vi "Show Open VIs Main Dialog.vi"(8 "error in (no error)":errorcluster) -> (0 "error out":errorcluster)   [LabVIEW 2011]
doc: "This VI will show a dialog of all the VIs that are currently open. Then this VI will allow you to select one to open the front panel, block diagram, or abort.\n\nDeveloped by Brian Hoover brian@brian-hoover.com"
uses:
  VI Data Type.ctl
  <vilib>/picture/picture.llb/imagedata.ctl
  <vilib>/Utility/miscctls.llb/LVBoundsTypeDef.ctl
  <userlib>/_OpenG.lib/array/array.llb/Conditional Auto-Indexing Tunnel (Variant)__ogtk.vi
  <userlib>/_OpenG.lib/file/file.llb/Strip Path - Traditional__ogtk.vi
panel:
  in  "n":dbl
  in  "Refresh":bool
  out "2D Picture":picture
  out "VI Name":string
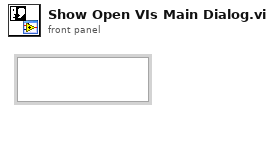
[diagram p1: front panel]
types:
  T1 = typedef "LVBoundsTypeDef.ctl" = cluster{"Width":u32, "Height":u32}
  T2 = typedef "VI Data Type.ctl" = cluster{"App Refnum":refnum<vi>, "VI Name":string, "VI Icon":T3}
  T3 = typedef "imagedata.ctl" = cluster{"image type":i32, "image depth":i32, "image":u8[], "mask":u8[], "colors":u32[], "Rectangle":cluster{"left":i16, "top":i16, "right":i16, "bottom":i16}}
  T4 = cluster{"Resize?":bool, "All VI Data":T2[], "Last Selected VI":T2, "Cell Bounds":T1, "# of Rows":i32, "# of Columns":i32, "Original Picture":picture}
  T5 = cluster{"Width":i16, "Style":enum32{"Solid", "Dash", "Dot", "DashDot", "DashDotDot"}}
  T6 = enum32{"Invalid", "Standard", "Closed", "Hidden", "Minimized", "Maximized"}
  T7 = typedef "LVPoint32TypeDef.ctl" = cluster{"Horizontal":i32, "Vertical":i32}
  T8 = cluster{"Width":u32, "Height":u32, "Width":u32, "Height":u32}
  T9 = cluster{"Shift":bool, "Ctrl":bool, "Alt":bool, "Cmd":bool, "Opt":bool}
  T10 = enum32{"Bad", "Idle", "Run top level", "Running"}
  T11 = typedef "VIMemory VI info.ctl" = cluster{"Project":string, "ComputingNode":string, "VI Name":string, "App Refnum":refnum<vi>}
  T12 = typedef "LVRectTypeDef.ctl" = cluster{"left":i16, "top":i16, "right":i16, "bottom":i16}
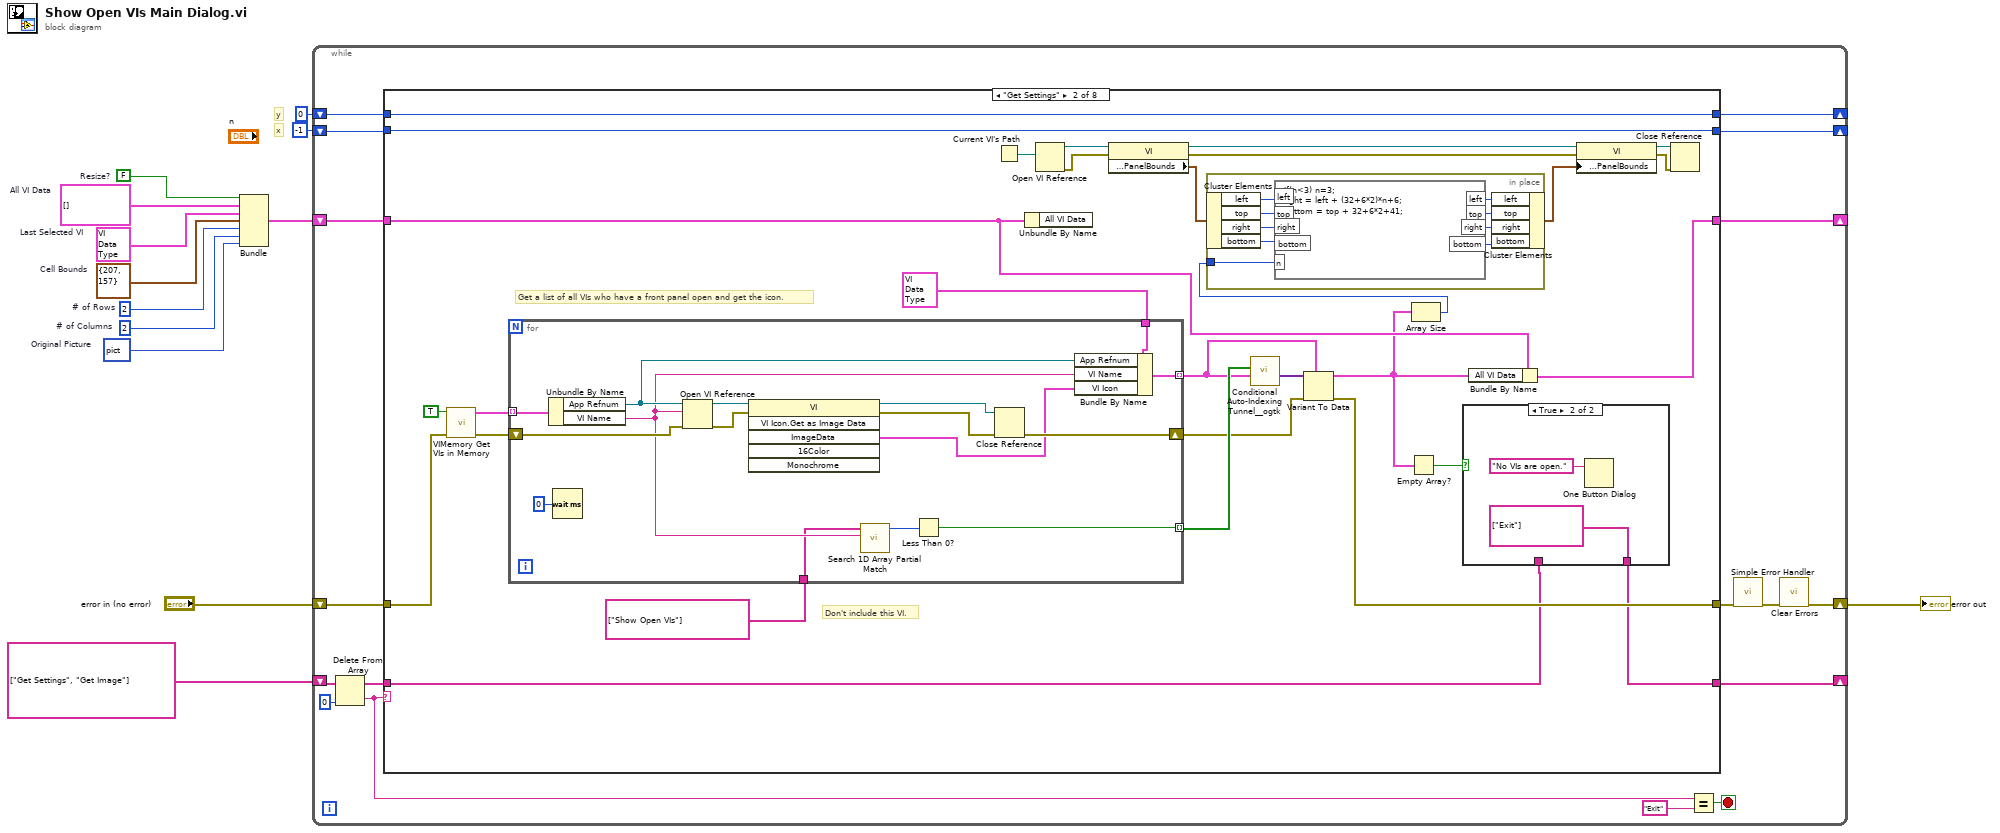
[diagram p0: block diagram]
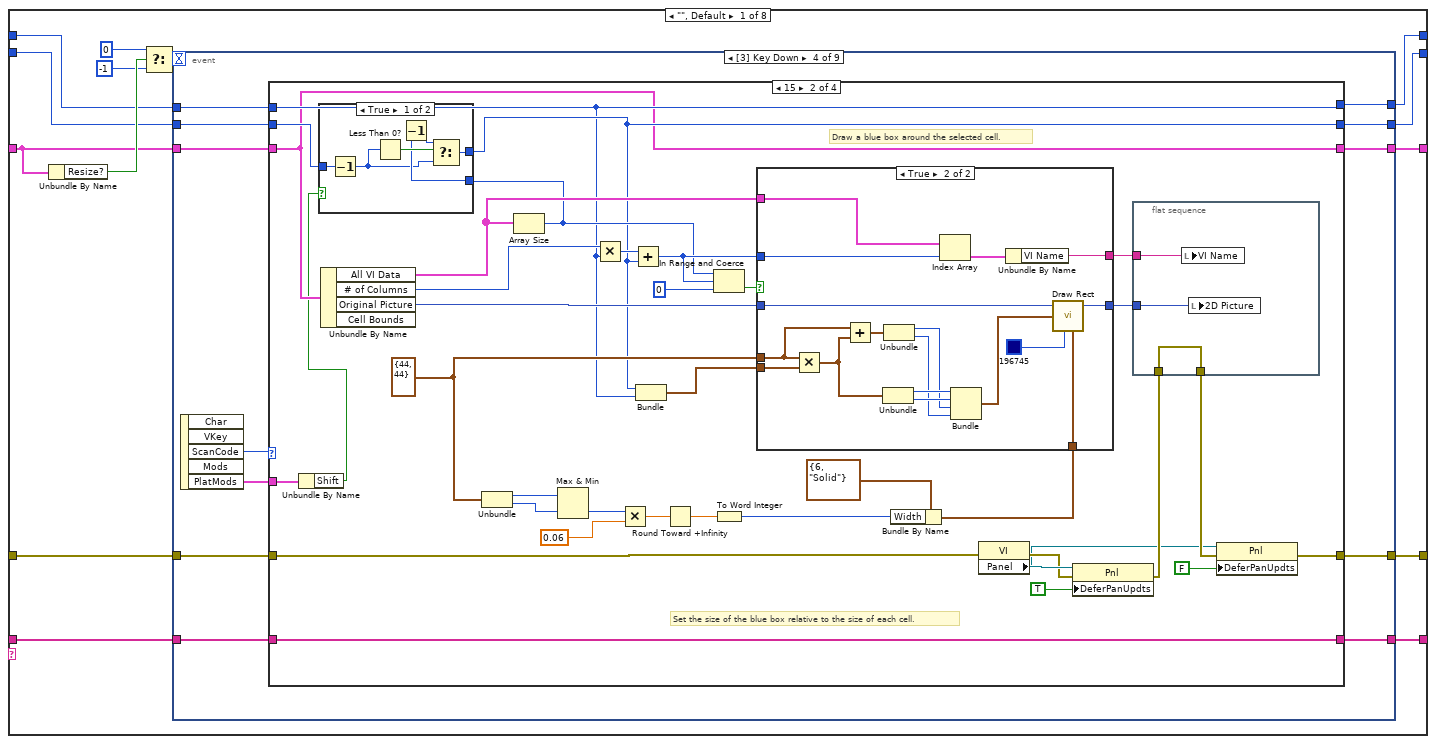
[diagram p2: hidden frame]
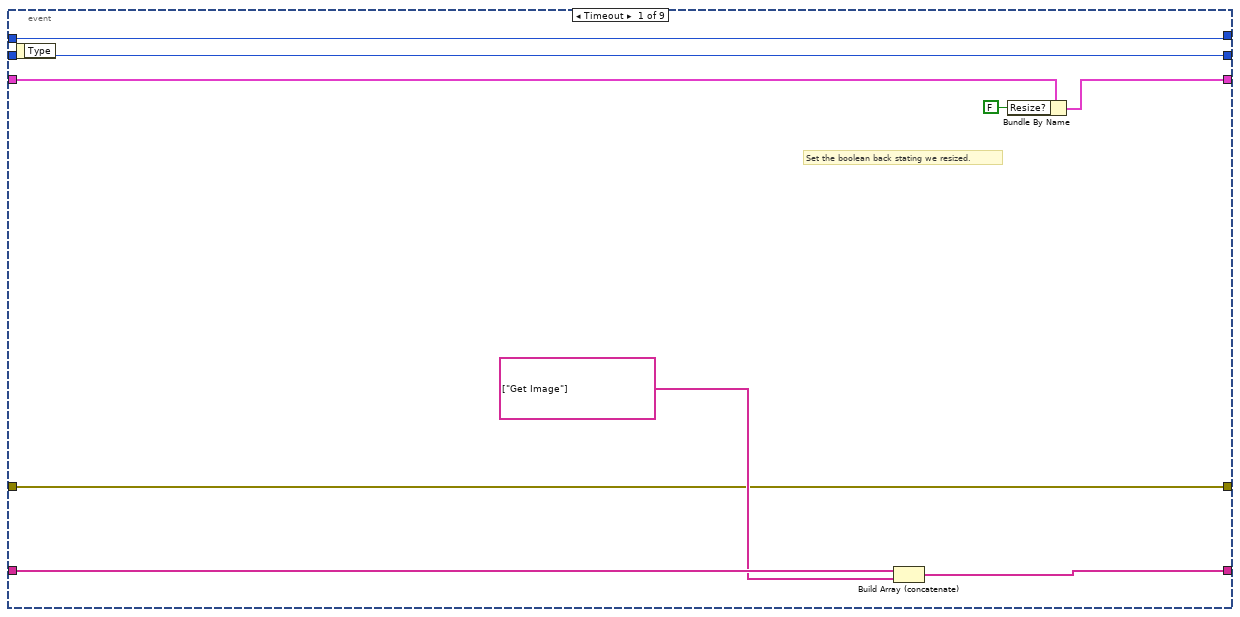
[diagram p3: hidden frame]
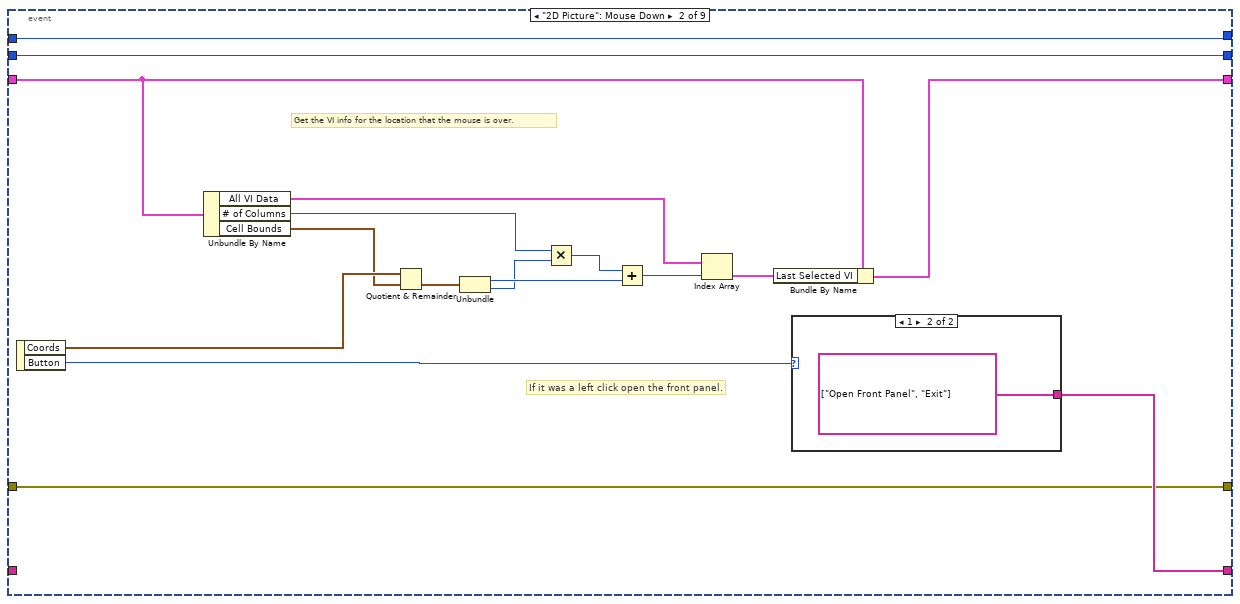
[diagram p4: hidden frame]
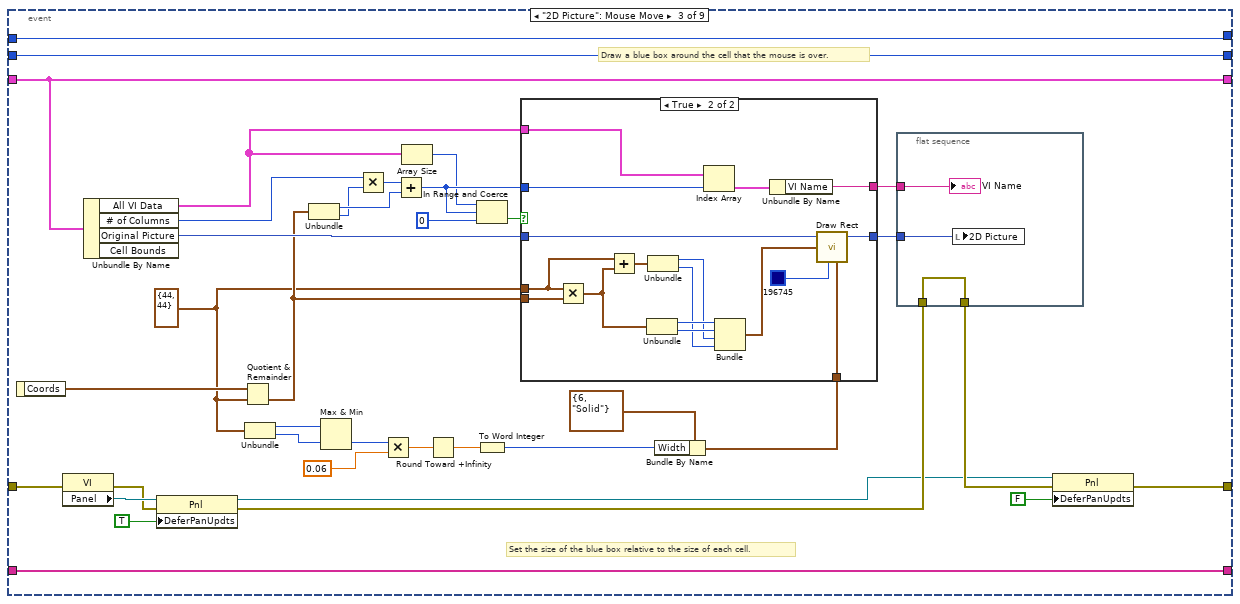
[diagram p6: hidden frame]
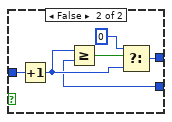
[diagram p9: hidden frame]
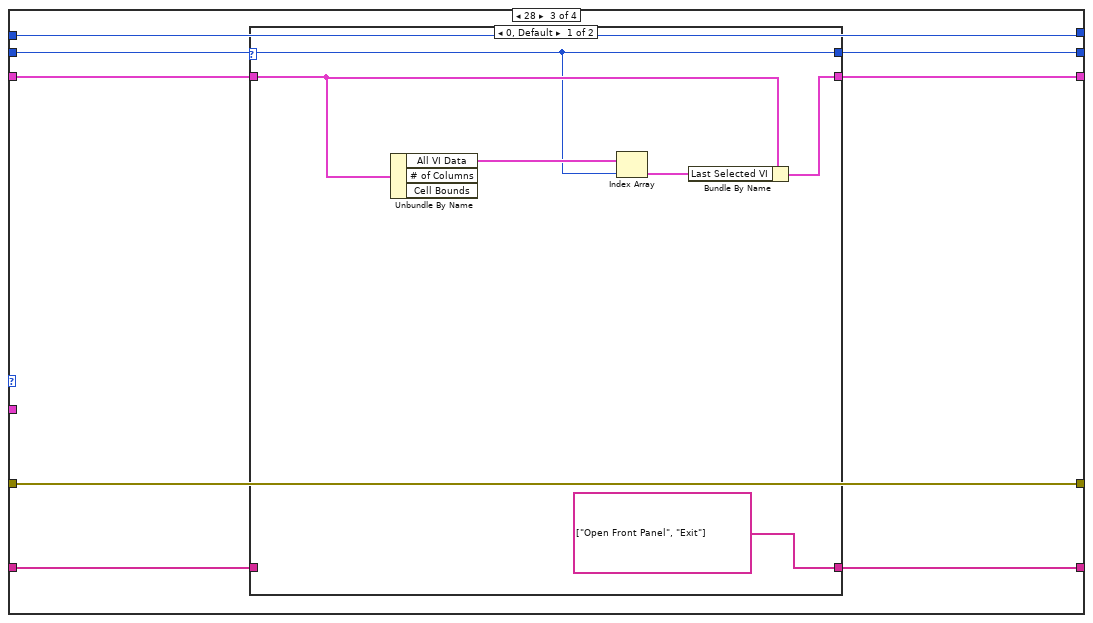
[diagram p11: hidden frame]
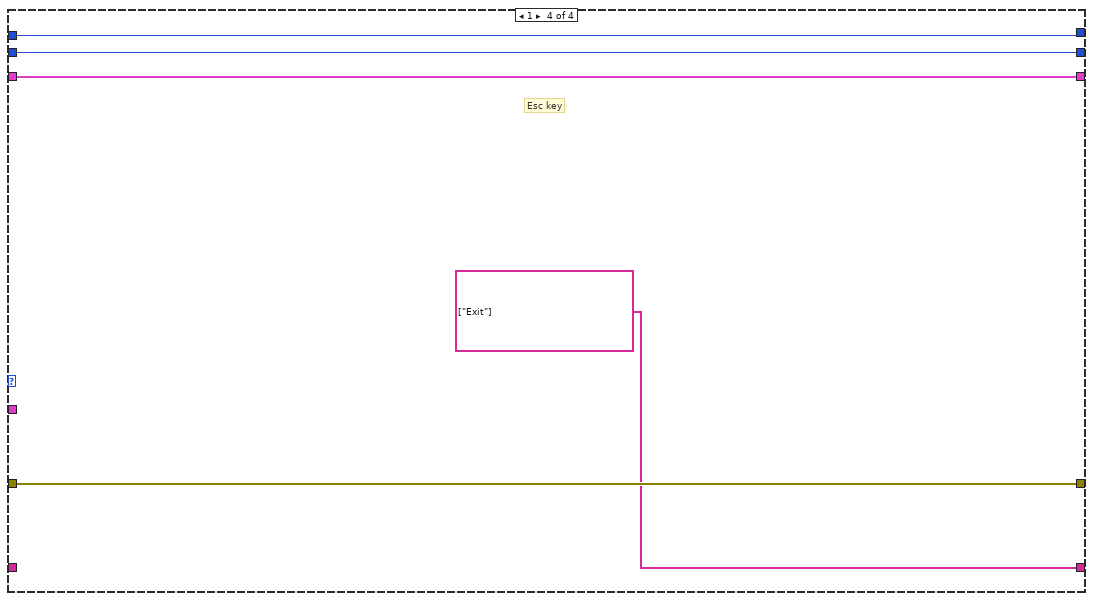
[diagram p13: hidden frame]
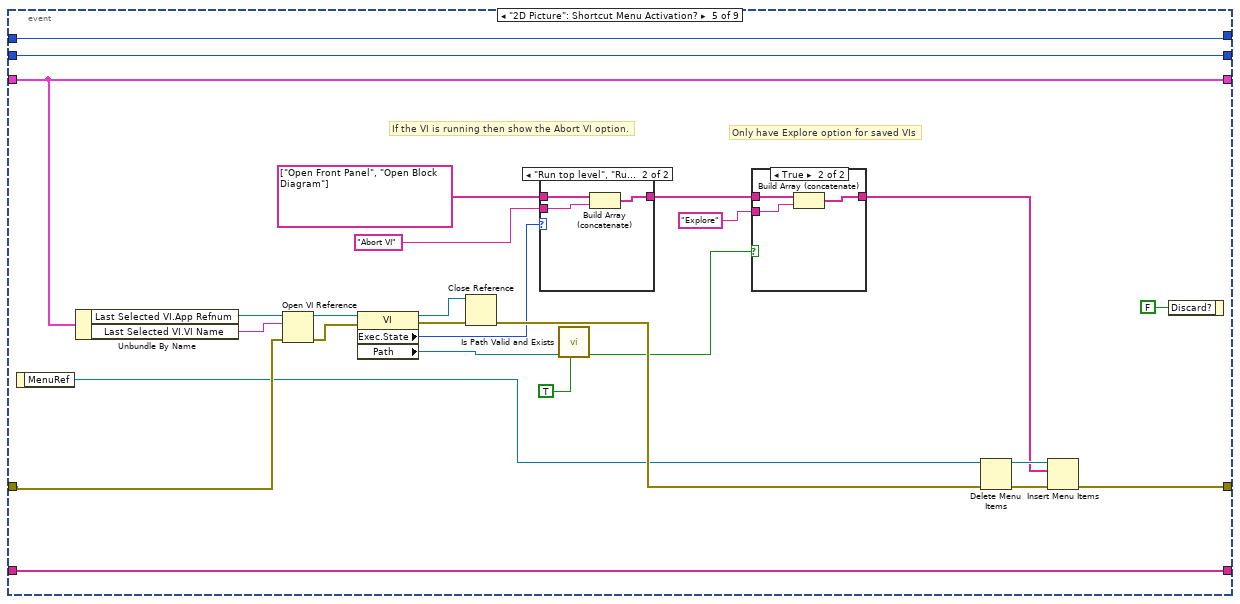
[diagram p14: hidden frame]
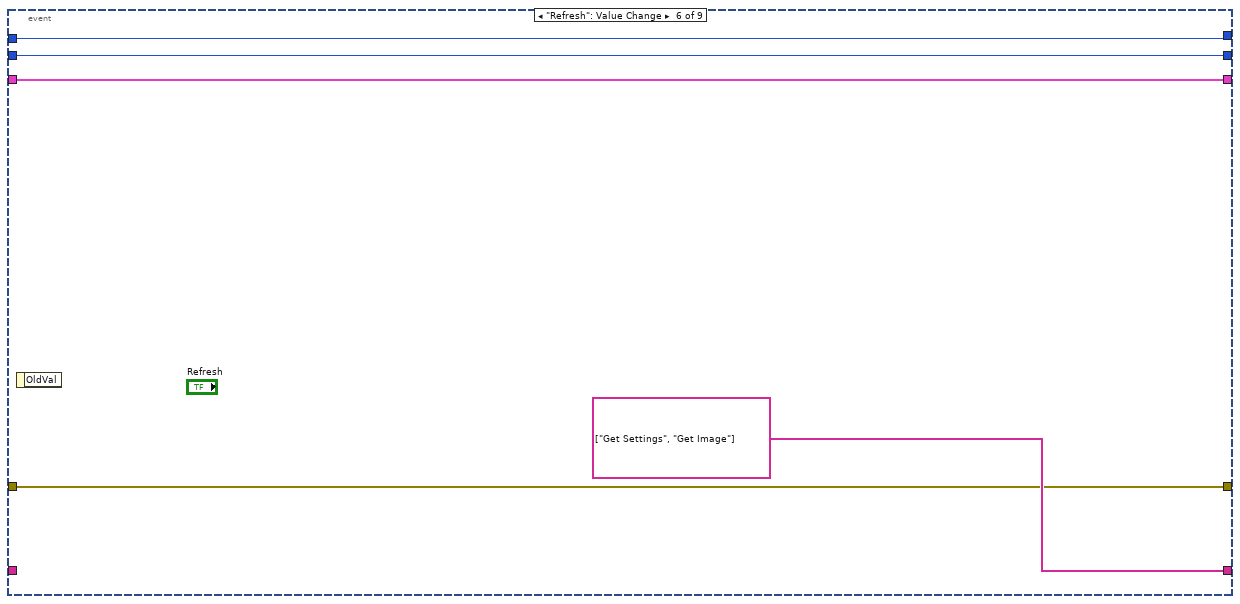
[diagram p17: hidden frame]
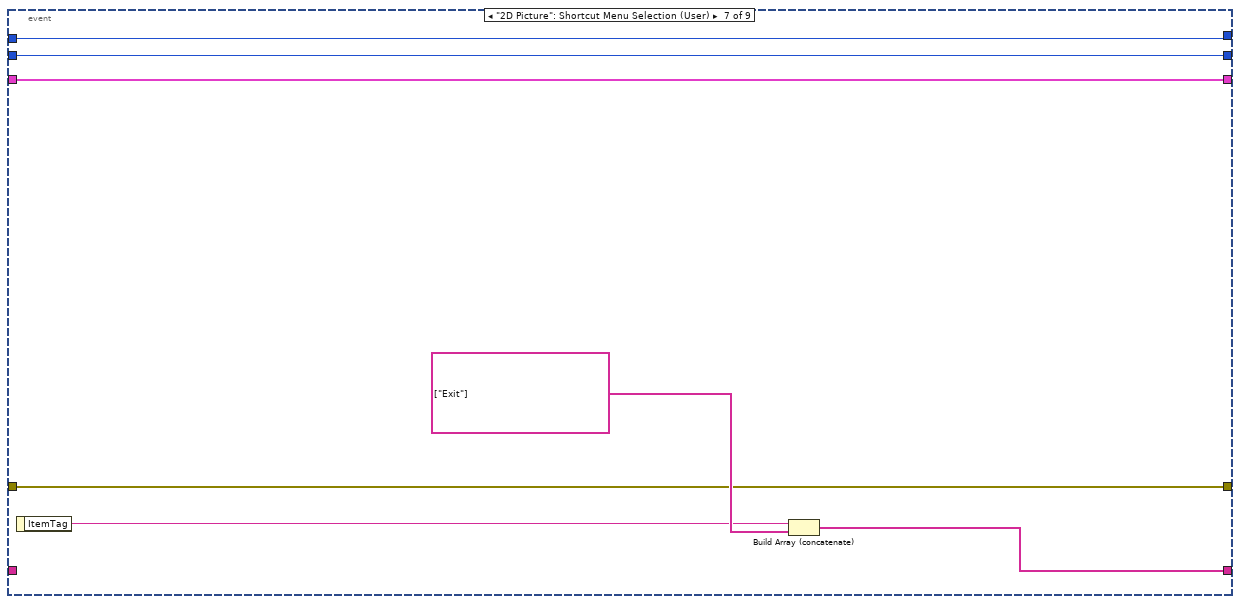
[diagram p18: hidden frame]
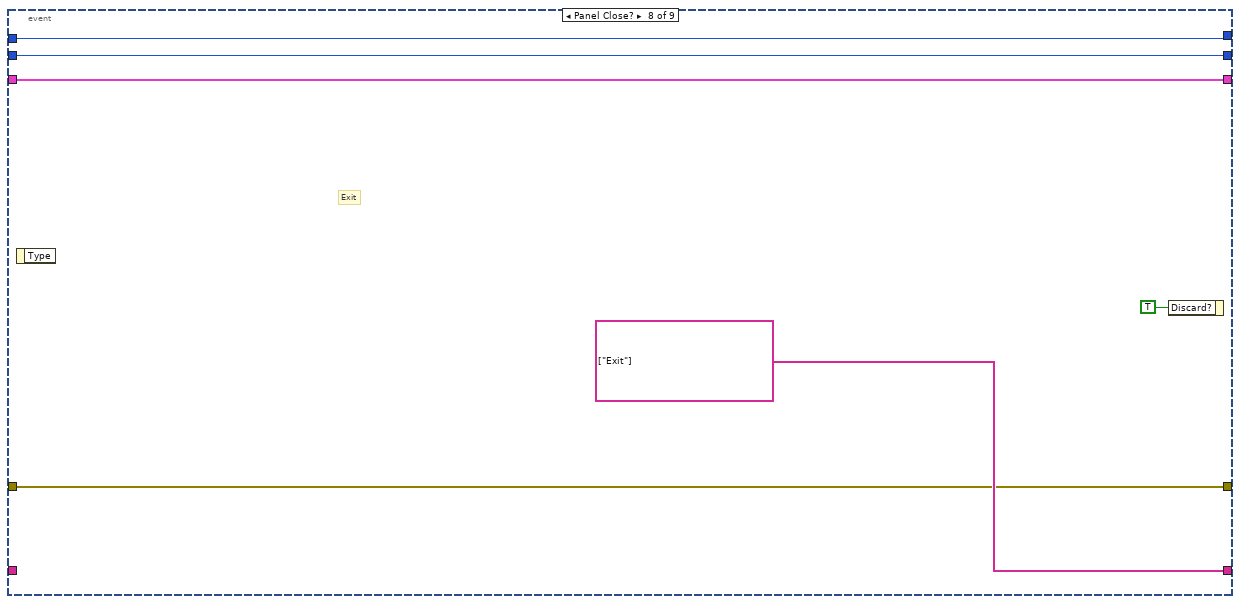
[diagram p19: hidden frame]
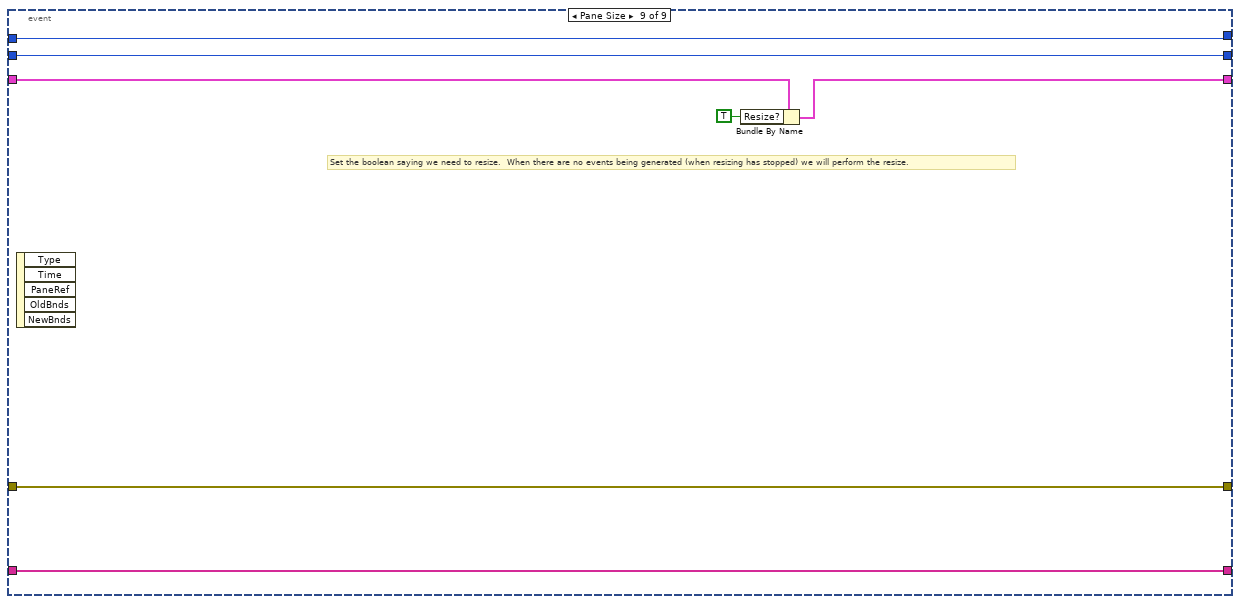
[diagram p20: hidden frame]
diagram:
  w3 = picture data[5B]  # Original Picture
  w4 = 2  # # of Columns
  w5 = 2  # # of Rows
  w6 = T1 {"Width"=207, "Height"=157}  # Cell Bounds
  w9 = T2 {"App Refnum"=refnum, "VI Name"="", "VI Icon"={"image type"=0, "image depth"=0, "image"=[], "mask"=[], "colors"=[], "Rectangle"={"left"=0, "top"=0, "right"=0, "bottom"=0}}}  # Last Selected VI
  w10 = T2[] []  # All VI Data
  w11 = FALSE  # Resize?
  # "y"
  # "x"
  n1 = Bundle("Resize?"=w11, "All VI Data"=w10, "Last Selected VI"=w9, "Cell Bounds"=w6, "# of Rows"=w5, "# of Columns"=w4, "Original Picture"=w3) -> (w12:T4)  [unwired: 1 in]
  n2 = while {
    shift-right: [w26] -> _
    shift-left: string[] ["Get Settings", "Get Image"] -> [w29]
    shift-right: [w22] -> _
    shift-left: w12 -> [w23]
    shift-right: [w19] -> w7
    shift-left: "error in (no error)" -> [w21]
    shift-right: [w16] -> _
    shift-left: -1 -> [w17]
    shift-right: [w15] -> _
    shift-left: 0 -> [w14]
    stop <- w30 stop-if-true
    n3 = Delete From Array(array=w29, index=0) -> (deleted portion=w28:string, array with subset deleted=w27:string[])  [unwired: 1 in]
    n4 = case shown="\"Get Settings\"" w28 {
      tunnel: w27 -> [w44 w313 w378 w394 w406 w419 w438 w449]
      tunnel: [w43 w312 w378 w394 w406 w419 w438 w449] -> w26
      tunnel: w23 -> [w35 w302 w366 w393 w405 w418 w437 w448]
      tunnel: [w42 w326 w364 w393 w405 w418 w437 w448] -> w22
      tunnel: w21 -> [w37 w315 w369 w384 w398 w410 w430 w447]
      tunnel: [w36 w316 w367 w383 w397 w409 w423 w447] -> w18
      tunnel: w17 -> [w34 w300 w356 w382 w396 w408 w421 w446]
      tunnel: [w33 w300 w356 w382 w396 w408 w421 w446] -> w16
      tunnel: w14 -> [w31 w299 w355 w381 w395 w407 w420 w445]
      tunnel: [w32 w299 w355 w381 w395 w407 w420 w445] -> w15
      frame "", Default {
        n5 = Unbundle By Name(w35) -> ("Resize?"=w41:bool)
        n6 = Select(t=0, s=w41, f=-1) -> (s? t:f=w39:i32)
        n7 = event shown="[3] Key Down" {
          selector: _ -> [_ _ _ _ _ _ _ _ _]
          dyn-events: _ -> [_ _ _ _ _ _ _ _ _]
          timeout: w39 -> [_ _ _ _ _ _ _ _ _]
          tunnel: w44 -> [w53 _ w73 w132 w241 _ _ _ w294]
          tunnel: [w49 w59 w73 w133 w241 string[] ["Get Settings", "Get Image"] w280 string[] ["Exit"] w294] -> w43
          tunnel: w35 -> [w50 w70 w107 w141 w256 w277 w284 w290 w297]
          tunnel: [w52 w62 w107 w131 w256 w277 w284 w290 w296] -> w42
          tunnel: w37 -> [w47 w56 w81 w140 w257 w275 w282 w287 w293]
          tunnel: [w47 w56 w78 w139 w254 w275 w282 w287 w293] -> w36
          tunnel: w34 -> [w46 w55 w74 w137 w240 w274 w279 w286 w292]
          tunnel: [w46 w55 w74 w136 w240 w274 w279 w286 w292] -> w33
          tunnel: w31 -> [w45 w54 w72 w135 w239 w273 w278 w285 w291]
          tunnel: [w45 w54 w72 w134 w239 w273 w278 w285 w291] -> w32
          event Timeout {
            # "Set the boolean back stating we resized."
            n8 = event-data() -> ()  [unwired: 1 in, 1 out]
            n9 = Build Array (concatenate)(w53, string[] ["Get Image"] ("array")) -> (w49:string[])
            n10 = Bundle By Name(cluster=w50, "Resize?"=FALSE) -> (w52:T4)
          }
          event "2D Picture": Mouse Down {
            # "If it was a left click open the front panel."
            # "Get the VI info for the location that the mouse is over."
            n11 = event-data() -> ("Coords"=w69:T7, "Button"=w60:u16)  [unwired: 1 in]
            n12 = Unbundle By Name(w70) -> ("All VI Data"=w64:T2[], "# of Columns"=w66:i32, "Cell Bounds"=w68:T1)
            n13 = Quotient & Remainder(x=w69, y=w68) -> (floor(x/y)=w67:T1)  [unwired: 1 out]
            n14 = Unbundle(w67) -> ("Width"=w58:u32, "Height"=w57:u32)
            n15 = Multiply(x=w66, y=w57) -> (x*y=w65:u32)
            n16 = Add(x=w65, y=w58) -> (x+y=w63:u32)
            n17 = Index Array(array=w64, index=w63) -> (element=w61:T2)
            n18 = Bundle By Name(cluster=w70, "Last Selected VI"=w61) -> (w62:T4)
            n19 = case shown="1" w60 {
              tunnel: [_ string[] ["Open Front Panel", "Exit"]] -> w59
              frame 0, Default {
              }
              frame 1 {
              }
            }
          }
          event "2D Picture": Mouse Move {
            w75 = T1 {"Width"=44, "Height"=44} ("Cell Bounds")
            # "Draw a blue box around the cell that the mouse is over."
            # "Set the size of the blue box relative to the size of each cell."
            n20 = event-data() -> ("Coords"=w108:T7)  [unwired: 1 in]
            n21 = property class="VI"(error in=w81) -> (error out=w82:errorcluster, "Panel"=w84:refnum<vi>)  [unwired: 1 in, 1 out]
            n22 = Unbundle By Name(w107) -> ("All VI Data"=w90:T2[], "# of Columns"=w102:i32, "Original Picture"=w106:picture)  [unwired: 1 out]
            n23 = property class="Pnl"(reference=w84, error in=w82, "DeferPanUpdts"=TRUE ("Defer Panel Updates? (F)")) -> (reference out=w76:refnum<vi>, error out=w80:errorcluster)
            n24 = Quotient & Remainder(x=w108, y=w75) -> (floor(x/y)=w101:T1)  [unwired: 1 out]
            n25 = Unbundle(w75) -> ("Width"=w100:u32, "Height"=w99:u32)
            n26 = Unbundle(w101) -> ("Width"=w86:u32, "Height"=w85:u32)
            n27 = Max & Min(x=w100, y=w99) -> (min(x,y)=w98:u32)  [unwired: 1 out]
            n28 = Multiply(x=w102, y=w85) -> (x*y=w103:u32)
            n29 = Multiply(x=w98, y=0.06) -> (x*y=w97:dbl)
            n30 = Add(x=w103, y=w86) -> (x+y=w91:u32)
            n31 = Array Size(array=w90) -> (size(s)=w89:i32)
            n32 = Round Toward +Infinity(x=w97) -> (ceil(x): smallest int >= x=w95:dbl)
            n33 = In Range and Coerce(upper limit=w89, x=w91, lower limit=u32 0) -> (In Range?=w87:bool)  [unwired: 1 out]
            n34 = To Word Integer(number=w95) -> (16bit integer=w94:i16)
            n35 = Bundle By Name(cluster=T5 {"Width"=6, "Style"=enum."Solid"} ("pen"), "Width"=w94) -> (w96:T5)
            n36 = case shown="True" w87 {
              tunnel: w106 -> [w112 w129]
              tunnel: [w112 w128] -> w104
              tunnel: w101 -> [_ w127]
              tunnel: w75 -> [_ w126]
              tunnel: w96 -> [_ w125]
              tunnel: w90 -> [_ w115]
              tunnel: w91 -> [_ w114]
              tunnel: [_ w113] -> w92
              frame False {
                # "Cell is outside the range, clear the blue box."
              }
              frame True {
                n37 = Multiply(x=w126, y=w127) -> (x*y=w122:T1)
                n38 = Add(x=w126, y=w122) -> (x+y=w123:T1)
                n39 = Unbundle(w122) -> ("Width"=w121:u32, "Height"=w120:u32)
                n40 = Unbundle(w123) -> ("Width"=w119:u32, "Height"=w118:u32)
                n41 = Index Array(array=w115, index=w114) -> (element=w116:T2)
                n42 = Bundle("Width"=w121, "Height"=w120, "Width"=w119, "Height"=w118) -> (w117:T8)  [unwired: 1 in]
                n43 = Unbundle By Name(w116) -> ("VI Name"=w113:string)
                n44 = call <vilib>:"Draw Rect.vi"("picture"=w129, "rect"=w117, "color(black)"=u32 196745, "pen"=w125) -> ("new picture"=w128:picture)  [unwired: 5 in]
              }
            }
            n45 = flat-sequence {
              tunnel: w104 -> [w111]
              tunnel: w92 -> [w110]
              tunnel: w80 -> [w109]
              tunnel: [w109] -> w77
              frame #0 {
                n46 = local write "2D Picture"(w111) -> ()
                "VI Name" <- w110
              }
            }
            n47 = property class="Pnl"(reference=w76, error in=w77, "DeferPanUpdts"=FALSE ("Defer Panel Updates? (F)")) -> (error out=w78:errorcluster)  [unwired: 1 out]
          }
          event Key Down {
            n48 = event-data() -> ("ScanCode"=w138:i16, "PlatMods"=w130:T9)  [unwired: 1 in, 3 out]
            n49 = case shown="15" w138 {
              tunnel: w141 -> [w142 w149 w222 w238]
              tunnel: w140 -> [w146 w162 w224 w237]
              tunnel: [w146 w159 w224 w237] -> w139
              tunnel: w137 -> [w143 w155 w220 w236]
              tunnel: [w143 w153 w219 w236] -> w136
              tunnel: w135 -> [w145 w152 w223 w235]
              tunnel: [w145 w152 w223 w235] -> w134
              tunnel: [w144 w150 w217 string[] ["Exit"]] -> w133
              tunnel: w132 -> [w144 w150 w218 _]
              tunnel: [w142 w149 w221 w238] -> w131
              tunnel: w130 -> [_ w148 _ _]
              frame 0, Default {
                # "Ignore other keys"
              }
              frame 15 {
                w156 = T1 {"Width"=44, "Height"=44} ("Cell Bounds")
                # "Draw a blue box around the selected cell."
                # "Set the size of the blue box relative to the size of each cell."
                n50 = Unbundle By Name(w148) -> ("Shift"=w147:bool)
                n51 = Unbundle By Name(w149) -> ("All VI Data"=w168:T2[], "# of Columns"=w179:i32, "Original Picture"=w183:picture)  [unwired: 1 out]
                n52 = Unbundle(w156) -> ("Width"=w178:u32, "Height"=w177:u32)
                n53 = Array Size(array=w168) -> (size(s)=w154:i32)
                n54 = case shown="True" w147 {
                  tunnel: w155 -> [w189 w195]
                  tunnel: w154 -> [w185 w191]
                  tunnel: [w187 w190] -> w153
                  frame True {
                    n55 = Decrement(x=w189) -> (x-1=w184:i32)
                    n56 = Less Than 0?(x=w184) -> (x < 0?=w188:bool)
                    n57 = Decrement(x=w185) -> (x-1=w186:i32)
                    n58 = Select(t=w186, s=w188, f=w184) -> (s? t:f=w187:i32)
                  }
                  frame False {
                    n59 = Increment(x=w195) -> (x+1=w192:i32)
                    n60 = Greater Or Equal?(x=w192, y=w191) -> (x >= y?=w194:bool)
                    n61 = Select(t=0, s=w194, f=w192) -> (s? t:f=w190:i32)
                  }
                }
                n62 = Max & Min(x=w178, y=w177) -> (min(x,y)=w176:u32)  [unwired: 1 out]
                n63 = Multiply(x=w179, y=w152) -> (x*y=w180:i32)
                n64 = Multiply(x=w176, y=0.06) -> (x*y=w175:dbl)
                n65 = Add(x=w180, y=w153) -> (x+y=w169:i32)
                n66 = Bundle(w153, w152) -> (w151:cluster{i32, i32})  [unwired: 1 in]
                n67 = Round Toward +Infinity(x=w175) -> (ceil(x): smallest int >= x=w173:dbl)
                n68 = In Range and Coerce(upper limit=w154, x=w169, lower limit=u32 0) -> (In Range?=w166:bool)  [unwired: 1 out]
                n69 = To Word Integer(number=w173) -> (16bit integer=w172:i16)
                n70 = Bundle By Name(cluster=T5 {"Width"=6, "Style"=enum."Solid"} ("pen"), "Width"=w172) -> (w174:T5)
                n71 = case shown="True" w166 {
                  tunnel: w183 -> [w199 w216]
                  tunnel: [w199 w215] -> w181
                  tunnel: w151 -> [_ w214]
                  tunnel: w156 -> [_ w213]
                  tunnel: w174 -> [_ w212]
                  tunnel: w168 -> [_ w202]
                  tunnel: w169 -> [_ w201]
                  tunnel: [_ w200] -> w170
                  frame False {
                    # "Cell is outside the range, clear the blue box."
                  }
                  frame True {
                    n72 = Multiply(x=w213, y=w214) -> (x*y=w209:T1)
                    n73 = Add(x=w213, y=w209) -> (x+y=w210:T1)
                    n74 = Unbundle(w209) -> ("Width"=w208:u32, "Height"=w207:u32)
                    n75 = Unbundle(w210) -> ("Width"=w206:u32, "Height"=w205:u32)
                    n76 = Index Array(array=w202, index=w201) -> (element=w203:T2)
                    n77 = Bundle("Width"=w208, "Height"=w207, "Width"=w206, "Height"=w205) -> (w204:T8)  [unwired: 1 in]
                    n78 = Unbundle By Name(w203) -> ("VI Name"=w200:string)
                    n79 = call <vilib>:"Draw Rect.vi"("picture"=w216, "rect"=w204, "color(black)"=u32 196745, "pen"=w212) -> ("new picture"=w215:picture)  [unwired: 5 in]
                  }
                }
                n80 = property class="VI"(error in=w162) -> (error out=w163:errorcluster, "Panel"=w165:refnum<vi>)  [unwired: 1 in, 1 out]
                n81 = property class="Pnl"(reference=w165, error in=w163, "DeferPanUpdts"=TRUE ("Defer Panel Updates? (F)")) -> (reference out=w157:refnum<vi>, error out=w161:errorcluster)
                n82 = flat-sequence {
                  tunnel: w181 -> [w198]
                  tunnel: w170 -> [w196]
                  tunnel: w161 -> [w197]
                  tunnel: [w197] -> w158
                  frame #0 {
                    n83 = local write "VI Name"(w196) -> ()
                    n84 = local write "2D Picture"(w198) -> ()
                  }
                }
                n85 = property class="Pnl"(reference=w157, error in=w158, "DeferPanUpdts"=FALSE ("Defer Panel Updates? (F)")) -> (error out=w159:errorcluster)  [unwired: 1 out]
              }
              frame 28 {
                n86 = case shown="0, Default" w220 {
                  selector: w220 -> [w226 w231]
                  tunnel: w222 -> [w228 w232]
                  tunnel: [w227 w232] -> w221
                  tunnel: [w226 w231] -> w219
                  tunnel: w218 -> [_ w233]
                  tunnel: [string[] ["Open Front Panel", "Exit"] w233] -> w217
                  frame 0, Default {
                    n87 = Unbundle By Name(w228) -> ("All VI Data"=w230:T2[])  [unwired: 2 out]
                    n88 = Index Array(array=w230, index=w226) -> (element=w229:T2)
                    n89 = Bundle By Name(cluster=w228, "Last Selected VI"=w229) -> (w227:T4)
                  }
                  frame -1 {
                    # "If nothing is selected, do nothing."
                  }
                }
              }
              frame 1 {
                # "Esc key"
              }
            }
          }
          event "2D Picture": Shortcut Menu Activation? {
            # "Only have Explore option for saved VIs"
            # "If the VI is running then show the Abort VI option."
            n90 = event-data() -> ("MenuRef"=w255:refnum<k9>)  [unwired: 1 in]
            n91 = Unbundle By Name(w256) -> ("Last Selected VI.App Refnum"=w264:refnum<vi>, "Last Selected VI.VI Name"=w263:string)
            n92 = Open VI Reference(application reference (local)=w264, vi path=w263, error in (no error)=w257) -> (vi reference=w262:refnum<vi>, error out=w259:errorcluster)  [unwired: 3 in]
            n93 = property class="VI"(reference=w262, error in=w259) -> (reference out=w261:refnum<vi>, error out=w260:errorcluster, "Exec.State"=w252:T10, "Path"=w246:path)
            n94 = Close Reference(reference=w261, error in (no error)=w260) -> (error out=w258:errorcluster)
            n95 = case shown="\"Run top level\", \"Running\"" w252 {
              tunnel: string[] ["Open Front Panel", "Open Block Diagram"] ("item names") -> [w269 w272]
              tunnel: "Abort VI" -> [_ w271]
              tunnel: [w269 w270] -> w247
              frame Default {
              }
              frame "Run top level", "Running" {
                n96 = Build Array (concatenate)(w272, w271) -> (w270:string[])
              }
            }
            n97 = call "Is Path Valid and Exists.vi"("Check Inside LLBs?"=TRUE, "File/Folder Path"=w246) -> ("Valid and Exists?"=w245:bool)  [unwired: 8 in, 1 out]
            n98 = case shown="True" w245 {
              tunnel: w247 -> [w265 w268]
              tunnel: "Explore" -> [_ w267]
              tunnel: [w265 w266] -> w244
              frame False {
              }
              frame True {
                n99 = Build Array (concatenate)(w268, w267) -> (w266:string[])
              }
            }
            n100 = Delete Menu Items(6:w258, 9:w255) -> (0:w249:errorcluster, 3:w248:refnum<k9>)  [unwired: 2 in]
            n101 = Insert Menu Items(6:w249, 8:w244, 9:w248) -> (0:w254:errorcluster)  [unwired: 3 in, 2 out]
            n102 = event-data("Discard?"=FALSE) -> ()  [unwired: 1 in, 1 out]
          }
          event "Refresh": Value Change {
            n103 = event-data() -> ()  [unwired: 1 in, 1 out]
          }
          event "2D Picture": Shortcut Menu Selection (User) {
            n104 = event-data() -> ("ItemTag"=w281:string)  [unwired: 1 in]
            n105 = Build Array (concatenate)(w281, string[] ["Exit"]) -> (w280:string[])
          }
          event Panel Close? {
            # "Exit"
            n106 = event-data() -> ()  [unwired: 1 in, 1 out]
            n107 = event-data("Discard?"=TRUE) -> ()  [unwired: 1 in, 1 out]
          }
          event Pane Size {
            # "Set the boolean saying we need to resize.  When there are no events being generated (when resizing has stopped) we will perform the resize."
            n108 = event-data() -> ()  [unwired: 1 in, 5 out]
            n109 = Bundle By Name(cluster=w297, "Resize?"=TRUE) -> (w296:T4)
          }
        }
      }
      frame "Get Settings" {
        # "Get a list of all VIs who have a front panel open and get the icon."
        # "Don't include this VI."
        n110 = call <vilib>:"VIMemory Get VIs in Memory.vi"("error in (no error)"=w315, "Only VIs with Open FPs?"=TRUE) -> ("error out"=w323:errorcluster, "VIs in memory"=w324:T11[])  [unwired: 8 in]
        n111 = for {
          tunnel: w324 -> [w354] mode=indexing
          shift-right: [w352] -> w317
          shift-left: w323 -> [w353]
          tunnel: T2 {"App Refnum"=refnum, "VI Name"="", "VI Icon"={"image type"=0, "image depth"=0, "image"=[], "mask"=[], "colors"=[], "Rectangle"={"left"=0, "top"=0, "right"=0, "bottom"=0}}} ("VI Data") -> [w346]
          tunnel: [w344] -> w318 mode=indexing
          tunnel: string[] ["Show Open VIs"] ("1D array") -> [w341]
          tunnel: [w339] -> w319 mode=indexing
          n112 = Unbundle By Name(w354) -> ("App Refnum"=w345:refnum<vi>, "VI Name"=w342:string)
          n113 = Wait (ms)(milliseconds to wait=u32 0) -> ()  [unwired: 1 out]
          n114 = Open VI Reference(application reference (local)=w345, vi path=w342, error in (no error)=w353) -> (vi reference=w351:refnum<vi>, error out=w350:errorcluster)  [unwired: 3 in]
          n115 = invoke class="VI" method="VI Icon.Get as Image Data"(reference=w351, error in=w350) -> (reference out=w349:refnum<vi>, error out=w348:errorcluster, "ImageData"=w343:T3)  [unwired: 4 in, 3 out]
          n116 = call "Search 1D Array Partial Match.vi"("Item to Search"=w342, "Search Strings"=w341) -> ("First Index Found"=w340:i32)  [unwired: 9 in]
          n117 = Less Than 0?(x=w340) -> (x < 0?=w339:bool)
          n118 = Close Reference(reference=w349, error in (no error)=w348) -> (error out=w352:errorcluster)
          n119 = Bundle By Name(cluster=w346, "App Refnum"=w345, "VI Name"=w342, "VI Icon"=w343) -> (w344:T2)
        }
        n120 = Current VI's Path() -> (path=w309:path)
        n121 = Unbundle By Name(w302) -> ()  [unwired: 1 out]
        n122 = Open VI Reference(vi path=w309) -> (vi reference=w308:refnum<vi>, error out=w307:errorcluster)  [unwired: 5 in]
        n123 = property class="VI"(reference=w308, error in=w307) -> (reference out=w306:refnum<vi>, error out=w305:errorcluster, "Front Panel.PanelBounds"=w304:T12)
        n124 = call-poly <userlib>:"Conditional Auto-Indexing Tunnel__ogtk.vi"("Array in"=w318, "Elements to keep"=w319) -> ("Filtered Array out"=w320:variant[])  [unwired: 5 in]
        n125 = Variant To Data(error in=w317, type=w318, Variant=w320) -> (data=w298:T2[], error out=w316:errorcluster)
        n126 = Empty Array?(array=w298) -> (empty?=w314:bool)
        n127 = Array Size(array=w298) -> (size(s)=w301:i32)
        n128 = in-place {
          in-place-border: w301 -> [w327]
          n129 = in-place-cluster #1(w304) -> ("left"=w335:i16, "top"=w334:i16, "right"=w333:i16, "bottom"=w332:i16)
          n130 = formula code="if(n<3) n=3;\nright = left + (32+6*2)*n+6;\nbottom = top + 32+6*2+41;"("left"=w335, "top"=w334, "right"=w333, "bottom"=w332, "n"=w327) -> ("left"=w331:i16, "top"=w330:i16, "right"=w329:i16, "bottom"=w328:i16)
          n131 = in-place-cluster #1("left"=w331, "top"=w330, "right"=w329, "bottom"=w328) -> (w303:T12)
        }
        n132 = case shown="True" w314 {
          tunnel: [w336 string[] ["Exit"] ("1D array")] -> w312
          tunnel: w313 -> [w336 _]
          frame False {
          }
          frame True {
            n133 = One Button Dialog(message="No VIs are open.") -> ()  [unwired: 1 in, 1 out]
          }
        }
        n134 = Bundle By Name(cluster=w302, "All VI Data"=w298) -> (w326:T4)
        n135 = property class="VI"(reference=w306, error in=w305, "Front Panel.PanelBounds"=w303) -> (reference out=w310:refnum<vi>, error out=w311:errorcluster)
        n136 = Close Reference(reference=w310, error in (no error)=w311) -> ()  [unwired: 1 out]
      }
      frame "Get Image" {
        # "Get the number of columns/rows, and the size of each item based on the panel size."
        n137 = property class="VI"(error in=w369) -> (error out=w368:errorcluster, "Panel"=w375:refnum<vi>)  [unwired: 1 in, 1 out]
        n138 = property class="Pnl"(reference=w375, error in=w368, "DeferPanUpdts"=TRUE ("Defer Panel Updates? (F)")) -> (reference out=w357:refnum<vi>, error out=w373:errorcluster)
        n139 = control-ref of="Pane"() -> (w365:refnum<vi>)
        n140 = Unbundle By Name(w366) -> ("All VI Data"=w370:T2[])
        n141 = property class="Pane"(reference=w365, error in=w373) -> (error out=w371:errorcluster, "Bounds"=w377:T1)  [unwired: 1 out]
        n142 = Array Size(array=w370) -> (size(s)=w376:i32)
        n143 = call "Calculate Number of Rows and Columns.vi"("# of items"=w376, "Bounds"=w377) -> ("# of Columns"=w361:i32, "# of Rows"=w362:i32, "Cell Bounds"=w363:T1)  [unwired: 7 in]
        n144 = call "Get Image Of VIs.vi"("# of Columns"=w361, "# of Rows"=w362, "error in (no error)"=w371, "Cell Bounds"=w363, "All VI Data"=w370) -> ("error out"=w359:errorcluster, "2D Picture"=w360:picture)  [unwired: 5 in]
        n145 = Bundle By Name(cluster=w366, "Cell Bounds"=w363, "# of Rows"=w362, "# of Columns"=w361, "Original Picture"=w360) -> (w364:T4)
        n146 = flat-sequence {
          tunnel: w360 -> [w380]
          tunnel: w359 -> [w379]
          tunnel: [w379] -> w358
          frame #0 {
            "2D Picture" <- w380
          }
        }
        n147 = property class="Pnl"(reference=w357, error in=w358, "DeferPanUpdts"=FALSE ("Defer Panel Updates? (F)")) -> (error out=w367:errorcluster)  [unwired: 1 out]
      }
      frame "Open Front Panel" {
        n148 = Unbundle By Name(w393) -> ("Last Selected VI.App Refnum"=w392:refnum<vi>, "Last Selected VI.VI Name"=w391:string)
        n149 = Open VI Reference(application reference (local)=w392, vi path=w391, error in (no error)=w384) -> (vi reference=w390:refnum<vi>, error out=w389:errorcluster)  [unwired: 3 in]
        n150 = invoke class="VI" method="FP.Open"(reference=w390, error in=w389, "Activate"=TRUE ("Activate?"), "State"=T6."Standard") -> (reference out=w386:refnum<vi>, error out=w385:errorcluster)  [unwired: 1 in, 3 out]
        n151 = Close Reference(reference=w386, error in (no error)=w385) -> (error out=w383:errorcluster)
      }
      frame "Abort VI" {
        n152 = Unbundle By Name(w405) -> ("Last Selected VI.App Refnum"=w404:refnum<vi>, "Last Selected VI.VI Name"=w403:string)
        n153 = Open VI Reference(application reference (local)=w404, vi path=w403, error in (no error)=w398) -> (vi reference=w402:refnum<vi>, error out=w401:errorcluster)  [unwired: 3 in]
        n154 = invoke class="VI" method="Abort VI"(reference=w402, error in=w401) -> (reference out=w400:refnum<vi>, error out=w399:errorcluster)  [unwired: 1 in, 1 out]
        n155 = Close Reference(reference=w400, error in (no error)=w399) -> (error out=w397:errorcluster)
      }
      frame "Open Block Diagram" {
        n156 = Unbundle By Name(w418) -> ("Last Selected VI.App Refnum"=w417:refnum<vi>, "Last Selected VI.VI Name"=w416:string)
        n157 = Open VI Reference(application reference (local)=w417, vi path=w416, error in (no error)=w410) -> (vi reference=w412:refnum<vi>, error out=w415:errorcluster)  [unwired: 3 in]
        n158 = property class="VI"(reference=w412, error in=w415, "BDWin.Open"=TRUE ("Block Diagram Window:Open")) -> (reference out=w414:refnum<vi>, error out=w413:errorcluster)
        n159 = Close Reference(reference=w414, error in (no error)=w413) -> (error out=w409:errorcluster)
      }
      frame "Explore" {
        # "Open the explorer window to the file."
        n160 = Unbundle By Name(w437) -> ("Last Selected VI.App Refnum"=w436:refnum<vi>, "Last Selected VI.VI Name"=w435:string)
        n161 = Open VI Reference(application reference (local)=w436, vi path=w435, error in (no error)=w430) -> (vi reference=w431:refnum<vi>, error out=w434:errorcluster)  [unwired: 3 in]
        n162 = property class="VI"(reference=w431, error in=w434) -> (reference out=w433:refnum<vi>, error out=w432:errorcluster, "Path"=w429:path)
        n163 = while {
          shift-right: [w439] -> w424
          shift-left: w429 -> [w441]
          stop <- w443 stop-if-true
          # "is Dir?"
          n164 = call-poly <userlib>:"Strip Path__ogtk.vi"("path"=w441) -> ("stripped path"=w439:path)  [unwired: 1 out]
          n165 = File/Directory Info(path=w439) -> (directory=w444:bool)  [unwired: 1 in, 6 out]
          n166 = Not A Number/Path/Refnum?(number/path/refnum=w441) -> (NaN/Path/Refnum?=w442:bool)
          n167 = Empty String/Path?(string/path=w441) -> (empty?=w440:bool)
          n168 = Compound Arithmetic op=OR(w444, w442, w440) -> (w443:bool)
        }
        n169 = Close Reference(reference=w433, error in (no error)=w432) -> (error out=w425:errorcluster)
        n170 = Format Into String(format string="cmd /c start explorer \"%s\"", w424) -> (resulting string=w428:string)  [unwired: 2 in, 1 out]
        n171 = call <vilib>:"System Exec.vi"("run minimized? (F)"=TRUE, "wait until completion? (T)"=FALSE, "error in (no error)"=w425, "command line"=w428) -> ("error out"=w423:errorcluster)  [unwired: 4 in, 3 out]
      }
      frame "Exit" {
      }
    }
    n172 = Equal?(x=w28, y="Exit") -> (x = y?=w30:bool)
    n173 = call <vilib>:"Simple Error Handler.vi"("error in (no error)"=w18) -> ("error out"=w20:errorcluster)  [unwired: 4 in, 4 out]
    n174 = call <vilib>:"Clear Errors.vi"("error in (no error)"=w20) -> ("error out"=w19:errorcluster)  [unwired: 6 in]
  }
  "error out" <- w7
